vi "Tracer_Level-Raw Data.vi"(6 "Calltree Level":i32, 8 "Error In":errorcluster, 9 "Data":string[](array[string])) -> (0 "Error Out":errorcluster)   [LabVIEW 2018, in "TracerLibrary.lvlib" / "Tracer.lvclass"]
uses:
  Tracer.lvclass
  protected/Tracer_ClassAttributes.vi
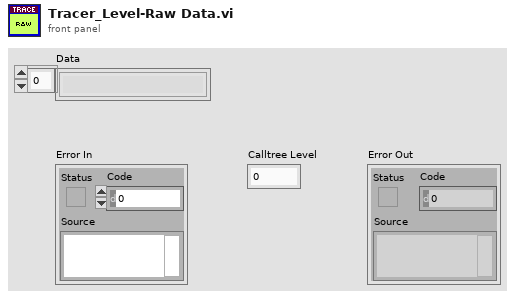
[diagram p1: front panel]
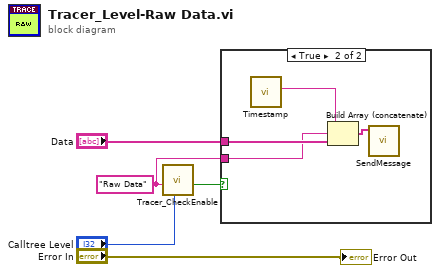
[diagram p0: block diagram]
diagram:
  w2 = "Raw Data" ("Category")
  n1 = call "Tracer_CheckEnable.vi"("Calltree Level"="Calltree Level", "Category"=w2) -> ("Trace Enabled"=w3:bool)  [unwired: 9 in]
  n2 = case shown="True" w3 {
    tunnel: "Data" -> [_ w7]
    tunnel: w2 -> [_ w6]
    frame False {
    }
    frame True {
      n3 = call "Timestamp.vi"() -> ("Date/time String"=w8:string)  [unwired: 11 in]
      n4 = Build Array (concatenate)(w8, w6, w7) -> (w9:string[])
      n5 = call "SendMessage.vi"("Msg"=w9) -> ()  [unwired: 11 in]
    }
  }
  "Error Out" <- "Error In"
